vi "Dataset Type 2 Transactions.vi"(10 "Dataset Type":T1, 11 "Sources":T3[](array[typedef])) -> (2 "Transactions":T2[](array[typedef]))   [LabVIEW 2013]
uses:
  Dataset Source.ctl
  Dataset Transaction Id.ctl
  Dataset Type.ctl
  Apps/Yes No Button.ctl
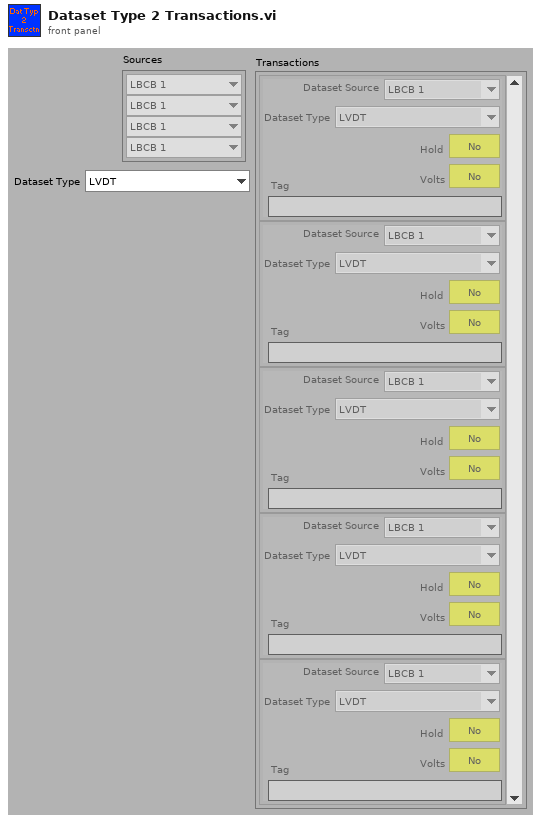
[diagram p1: front panel]
types:
  T1 = typedef "Dataset Type.ctl" = enum16{"LVDT", "Load Cell", "Actuator Command", "Servo Error", "Displacement Command", "Displacement", "Force"}
  T2 = typedef "Dataset Transaction Id.ctl" = cluster{"Dataset Source":T3, "Dataset Type":T1, "Hold":T4, "Volts":T4, "Tag":string}
  T3 = typedef "Dataset Source.ctl" = enum16{"LBCB 1", "LBCB 2", "Combined", "External Sensors"}
  T4 = typedef "Yes No Button.ctl" = bool
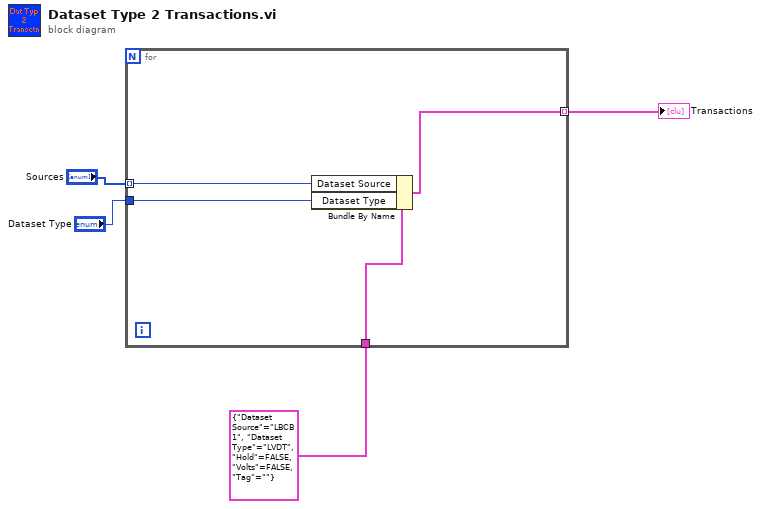
[diagram p0: block diagram]
diagram:
  n1 = for {
    tunnel: T2 {"Dataset Source"=enum."LBCB 1", "Dataset Type"=enum."LVDT", "Hold"=FALSE, "Volts"=FALSE, "Tag"=""} ("Dataset Trans Id") -> [w8]
    tunnel: "Sources" -> [w7] mode=indexing
    tunnel: "Dataset Type" -> [w6]
    tunnel: [w5] -> w1 mode=indexing
    n2 = Bundle By Name(cluster=w8, "Dataset Source"=w7, "Dataset Type"=w6) -> (w5:T2)
  }
  "Transactions" <- w1
